vi "01 - Syntax - Event API Syntax and Semantics.vi"() -> ()   [LabVIEW 2012]
panel:
  out "Tab Control":T1(tab)
  # "Jack Dunaway - CLA - LabVIEW Champion"
  # "Jack Dunaway - CLA - LabVIEW Champion"
  # "User Events Tips, Tricks, and Sundry"
  # "User Events Tips, Tricks, and Sundry"
  # "Follow along:"
  # "Follow along:"
  # "join.me/wirebirdlabs"
  # "join.me/wirebirdlabs"
  # "Download code:"
  # "Download code:"
  # "wirebird.co/CLA-Summit-2013-Paris"
  # "wirebird.co/CLA-Summit-2013-Paris"
  # "1. A Basic One-Click Deployment Automation Script\n\n2. Automating Inno Setup from the Command Line\n\n3. Uploading Application Installers to the web\n\n4. Creating a human-friendly Download Page for your customers\n\n5. Segmenting the Run-Time Engine and Dependencies for smaller installer footprint\n\n6. Use of Virgin Virtual Machines and Snapshots to test Deployments and End-User Experience\n\n7. You can open the webpage on your own computer and install this application!!"
  # "1. A Basic One-Click Deployment Automation Script\n\n2. Automating Inno Setup from the Command Line\n\n3. Uploading Application Installers to the web\n\n4. Creating a human-friendly Download Page for your customers\n\n5. Segmenting the Run-Time Engine and Dependencies for smaller installer footprint\n\n6. Use of Virgin Virtual Machines and Snapshots to test Deployments and End-User Experience\n\n7. You can open the webpage on your own computer and install this application!!"
  # "Agenda"
  # "Agenda"
  # "... the Ideal DevX:\nThe One-click deployment\n\n... the Ideal Customer Experience:\nThe Forehead Install"
  # "... the Ideal DevX:\nThe One-click deployment\n\n... the Ideal Customer Experience:\nThe Forehead Install"
  # "Goal: To approximate, or even achieve..."
  # "Goal: To approximate, or even achieve..."
  # "Inno Setup, free, open source setup authoring:\nhttp://www.jrsoftware.org/isinfo.php\n\nAmazon AWS SDK for .NET\nhttp://aws.amazon.com/sdkfornet/\n\nSegment the Run-Time Engine to minimize installer footprint:\nhttp://wirebird.co/Minify-RTE\n\nWirebird Labs Deploy: polished, powerful deployment automation\nhttps://wirebirdlabs.com/deploy"
  # "Inno Setup, free, open source setup authoring:\nhttp://www.jrsoftware.org/isinfo.php\n\nAmazon AWS SDK for .NET\nhttp://aws.amazon.com/sdkfornet/\n\nSegment the Run-Time Engine to minimize installer footprint:\nhttp://wirebird.co/Minify-RTE\n\nWirebird Labs Deploy: polished, powerful deployment automation\nhttps://wirebirdlabs.com/deploy"
  # "Links"
  # "Links"
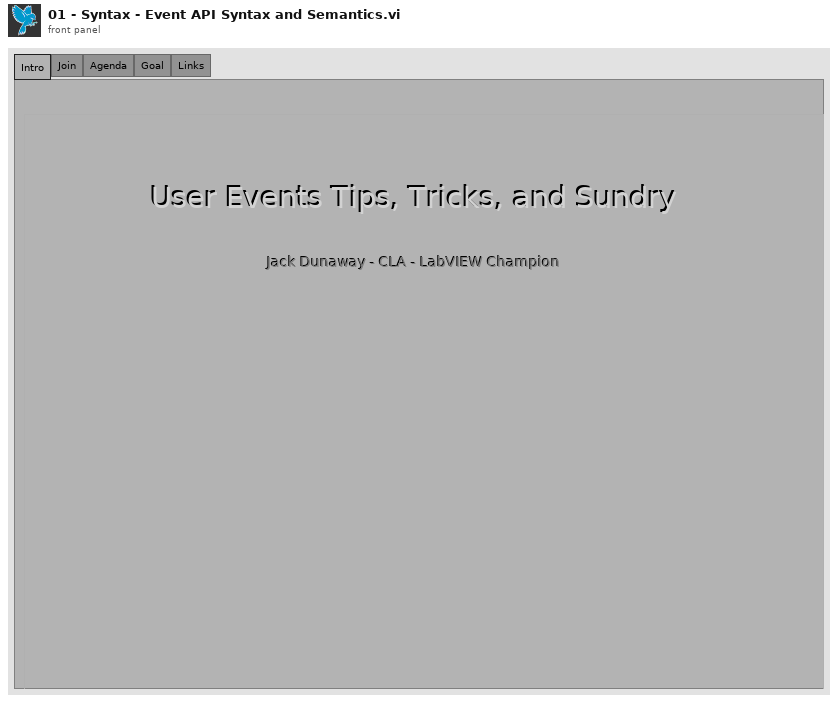
[diagram p1: front panel]
types:
  T1 = enum32{"Intro", "Join", "Agenda", "Goal", "Links"}
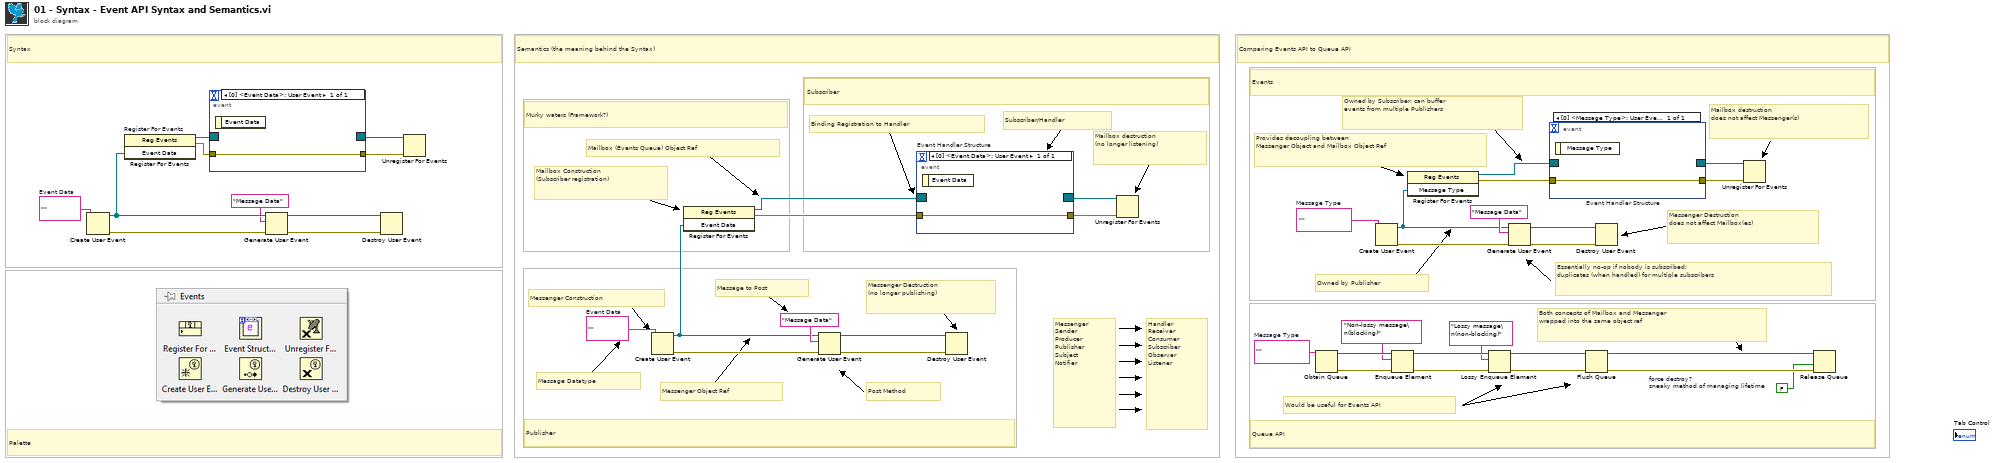
[diagram p0: block diagram]
diagram:
  w1 = ""  # Message Type
  w4 = FALSE  # force destroy? sneaky method of managing lifetime
  w18 = ""  # Message Type
  w28 = ""  # Event Data
  w37 = ""  # Event Data
  # "Would be useful for Events API"
  # "Both concepts of Mailbox and Messenger\nwrapped into the same object ref"
  # "Queue API"
  # "Events"
  # "Owned by Publisher"
  # "Comparing Events API to Queue API"
  # "Messenger Destruction\ndoes not affect Mailbox(es)"
  # "Mailbox destruction\ndoes not affect Messenger(s)"
  # "Essentially no-op if nobody is subscribed;\nduplicates (when handled) for multiple subscribers"
  # "Provides decoupling between\nMessenger Object and Mailbox Object Ref"
  # "Owned by Subscriber; can buffer\nevents from multiple Publishers"
  # "Messenger Object Ref"
  # "Message Datatype"
  # "Semantics (the meaning behind the Syntax)"
  # "Palette"
  # "Syntax"
  # "Messenger Destruction\n(no longer publishing)"
  # "Mailbox destruction\n(no longer listening)"
  # "Murky waters (Framework?)"
  # "Publisher"
  # "Subscriber"
  # "Post Method"
  # "Messenger Construction"
  # "Binding Registration to Handler"
  # "Handler\nReceiver\nConsumer\nSubscriber\nObserver\nListener"
  # "Messenger\nSender\nProducer\nPublisher\nSubject\nNotifier"
  # "Subscriber/Handler"
  # "Mailbox Construction\n(Subscriber registration)"
  # "Message to Post"
  # "Mailbox (Events Queue) Object Ref"
  n1 = Create User Event(user event datatype=w37) -> (user event=w41:refnum<user-event>, error out=w38:errorcluster)  [unwired: 1 in]
  n2 = register-events "Register For Events"(w41) -> (reference out=w42:refnum<event-registration>, error out=w35:errorcluster)  [unwired: 2 in]
  n3 = event shown="[0] <Event Data>: User Event" {
    selector: w42 -> [_]
    dyn-events: [_] -> w36
    timeout: _ -> [_]
    tunnel: w35 -> [w43]
    tunnel: [w43] -> w34
    event User Event {
      n4 = event-data() -> ()  [unwired: 1 in, 1 out]
    }
  }
  n5 = Generate User Event(user event=w41, event data cluster="Message Data" ("event data"), error in=w38) -> (user event out=w40:refnum<user-event>, error out=w39:errorcluster)
  n6 = Destroy User Event(user event=w40, error in=w39) -> ()  [unwired: 1 out]
  n7 = Unregister For Events(event registration refnum=w36, error in=w34) -> ()  [unwired: 1 out]
  n8 = Create User Event(user event datatype=w28) -> (user event=w24:refnum<user-event>, error out=w27:errorcluster)  [unwired: 1 in]
  n9 = register-events(w24) -> (reference out=w23:refnum<event-registration>, error out=w30:errorcluster)  [unwired: 2 in]
  n10 = Generate User Event(user event=w24, event data cluster="Message Data" ("event data"), error in=w27) -> (user event out=w25:refnum<user-event>, error out=w26:errorcluster)
  n11 = event "Event Handler Structure" shown="[0] <Event Data>: User Event" {
    selector: w23 -> [_]
    dyn-events: [_] -> w29
    timeout: _ -> [_]
    tunnel: w30 -> [w44]
    tunnel: [w44] -> w31
    event User Event {
      n12 = event-data() -> ()  [unwired: 1 in, 1 out]
    }
  }
  n13 = Destroy User Event(user event=w25, error in=w26) -> ()  [unwired: 1 out]
  n14 = Unregister For Events(event registration refnum=w29, error in=w31) -> ()  [unwired: 1 out]
  n15 = Obtain Queue(element data type=w1) -> (queue out=w12:refnum<queue>, error out=w11:errorcluster)  [unwired: 4 in, 1 out]
  n16 = Create User Event(user event datatype=w18) -> (user event=w14:refnum<user-event>, error out=w17:errorcluster)  [unwired: 1 in]
  n17 = Enqueue Element(queue=w12, element="Non-lossy message\n(blocking)", error in (no error)=w11) -> (queue out=w10:refnum<queue>, error out=w9:errorcluster)  [unwired: 1 in, 1 out]
  n18 = register-events(w14) -> (reference out=w13:refnum<event-registration>, error out=w20:errorcluster)  [unwired: 2 in]
  n19 = Lossy Enqueue Element(queue=w10, element="Lossy message\n(non-blocking)", error in (no error)=w9) -> (queue out=w7:refnum<queue>, error out=w8:errorcluster)  [unwired: 2 out]
  n20 = Generate User Event(user event=w14, event data cluster="Message Data" ("event data"), error in=w17) -> (user event out=w15:refnum<user-event>, error out=w16:errorcluster)
  n21 = event "Event Handler Structure" shown="[0] <Message Type>: User Event" {
    selector: w13 -> [_]
    dyn-events: [_] -> w19
    timeout: _ -> [_]
    tunnel: w20 -> [w45]
    tunnel: [w45] -> w21
    event User Event {
      n22 = event-data() -> ()  [unwired: 1 in, 1 out]
    }
  }
  n23 = Flush Queue(queue=w7, error in (no error)=w8) -> (queue out=w6:refnum<queue>, error out=w5:errorcluster)  [unwired: 1 out]
  n24 = Destroy User Event(user event=w15, error in=w16) -> ()  [unwired: 1 out]
  n25 = Unregister For Events(event registration refnum=w19, error in=w21) -> ()  [unwired: 1 out]
  n26 = Release Queue(queue=w6, force destroy? (F)=w4, error in (no error)=w5) -> ()  [unwired: 3 out]
